vi "Nested Malleable VIs - Lesson 2a.vi"() -> ()   [LabVIEW 2023]
doc: "Lesson 2 examines complex data types that have subtypes (such as arrays or clusters) and highlights how using a nesting level of VIM for each nested level of the data type can enable you to write complex algorithms that are easier to read and maintain."
uses:
  Equal Via Regular Expression Functor/Equal Via Regular Expression Functor.lvclass
  1a6d5e8e-a296-468e-9e55-2fb4af21a831.vi
  fd91f596-61ba-4296-af35-812e4d4f2264.vi
  d4cd4643-fb5c-4a6b-ac71-27e3804d891a.vi
  1a6d5e8e-a296-468e-9e55-2fb4af21a831.vi/5f008cf9-0835-42d5-ab12-715ade7a221f.vi
  fd91f596-61ba-4296-af35-812e4d4f2264.vi/5f008cf9-0835-42d5-ab12-715ade7a221f.vi
  1a6d5e8e-a296-468e-9e55-2fb4af21a831.vi/5f008cf9-0835-42d5-ab12-715ade7a221f.vi/4a937600-749b-4ff4-8f55-34e6a7c3203b.vi
  fd91f596-61ba-4296-af35-812e4d4f2264.vi/5f008cf9-0835-42d5-ab12-715ade7a221f.vi/4a937600-749b-4ff4-8f55-34e6a7c3203b.vi
  Equal Via Regular Expression Functor/Equals.vi
  <vilib>/Comparison/Equal/Equal Functor/Equal Functor.lvclass
panel:
  out "index of element 4":i32
  out "index of element 3":i32
  out "index of element 2":i32
  out "index of element 1":i32
  # "Overview: This lesson examines complex data types that have subtypes (such as arrays or clusters) and highlights how using another nesting level of VIM for each nested level of the data type can enable you to write complex algorithms that are easier to read and maintain.\n\nInstructions: \n1. Open the block diagram of this VI. Review the lessons presented there.\n2. Run the VI to see the results. \n3. Once you have finished reviewing this VI, open the next lesson VI in the Malleable VIs - Nested Malleable VIs example project."
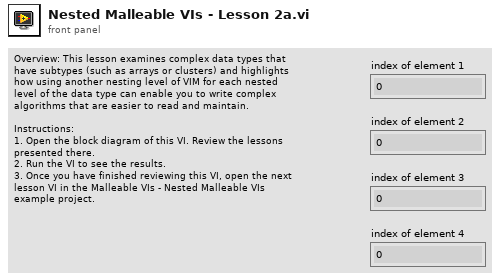
[diagram p1: front panel]
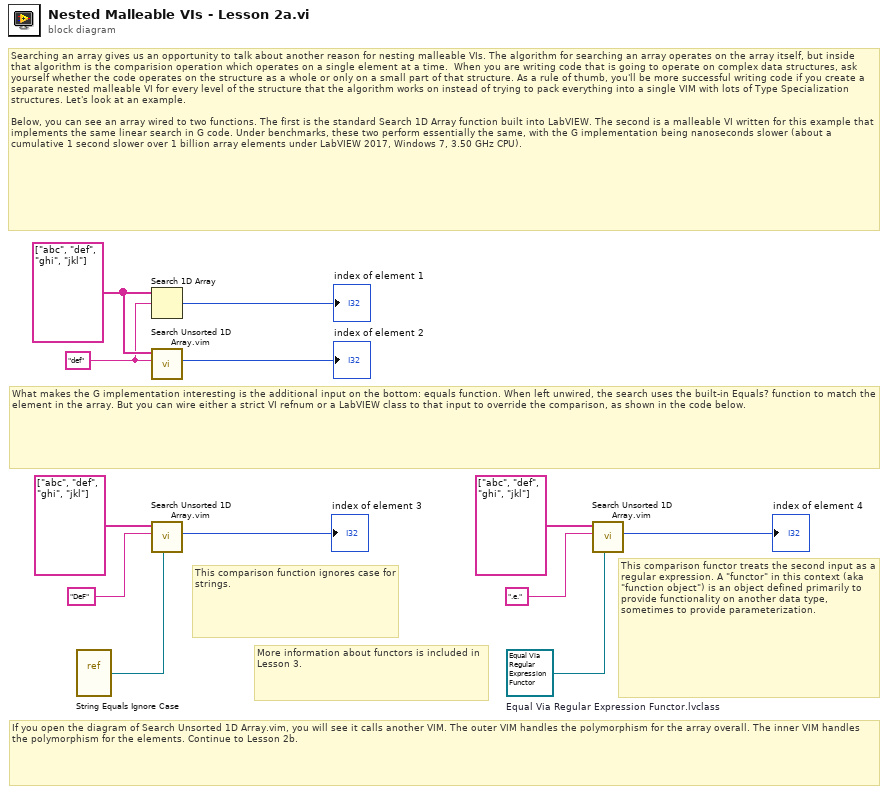
[diagram p0: block diagram]
diagram:
  w2 = refnum<class "Equal Via Regular Expression Functor.lvclass"> refnum  # Equal Via Regular Expression Functor.lvclass
  w9 = "def"
  w12 = string[] ["abc", "def", "ghi", "jkl"] ("1D array")
  # "More information about functors is included in Lesson 3."
  # "If you open the diagram of Search Unsorted 1D Array.vim, you will see it calls another VIM. The outer VIM handles the polymorphism for the array overall. The inner VIM handles the polymorphism for the elements. Continue to Lesson 2b."
  # "This comparison functor treats the second input as a regular expression. A \"functor\" in this context (aka \"function object\") is an object defined primarily to provide functionality on another data type, sometimes to provide parameterization."
  # "This comparison function ignores case for strings."
  # "What makes the G implementation interesting is the additional input on the bottom: equals function. When left unwired, the search uses the built-in Equals? function to match the element in the array. But you can wire either a strict VI refnum or a LabVIEW class to that input to override the comparison, as shown in the code below."
  # "Searching an array gives us an opportunity to talk about another reason for nesting malleable VIs. The algorithm for searching an array operates on the array itself, but inside that algorithm is the comparision operation which operates on a single element at a time.  When you are writing code that is going to operate on complex data structures, ask yourself whether the code operates on the structure as a whole or only on a small part of that structure. As a rule of thumb, you'll be more successful writing code if you create a separate nested malleable VI for every level of the structure that the algorithm works on instead of trying to pack everything into a single VIM with lots of Type Specialization structures. Let's look at an example.\n\nBelow, you can see an array wired to two functions. The first is the standard Search 1D Array function built into LabVIEW. The second is a malleable VI written for this example that implements the same linear search in G code. Under benchmarks, these two perform essentially the same, with the G implementation being nanoseconds slower (about a cumulative 1 second slower over 1 billion array elements under LabVIEW 2017, Windows 7, 3.50 GHz CPU)."
  n1 = vi-ref "String Equals Ignore Case.vi"() -> (w1:refnum<vi>)
  n2 = Search 1D Array(1D array=w12, element=w9) -> (index of element=→"index of element 1":i32)  [unwired: 1 in]
  n3 = call "Search Unsorted 1D Array.vim"("element"=w9, "unsorted 1D array"=w12) -> ("index of element"=→"index of element 2":i32)  [unwired: 9 in]
  n4 = call "Search Unsorted 1D Array.vim"("equals function (built-in =)"=w1, "element"="DeF", "unsorted 1D array"=string[] ["abc", "def", "ghi", "jkl"] ("1D array")) -> ("index of element"=→"index of element 3":i32)  [unwired: 8 in]
  n5 = call "Search Unsorted 1D Array.vim"("equals function (built-in =)"=w2, "element"=".e.", "unsorted 1D array"=string[] ["abc", "def", "ghi", "jkl"] ("1D array")) -> ("index of element"=→"index of element 4":i32)  [unwired: 8 in]
